vi "Set_Decoration_Color.vi"(0 "Pane ref":refnum<vi>, 5 "Data In":T1, 9 "Display State In":T2={"State 1"={"BG"=0, "FG"=0}, "State 0"={"BG"=0, "FG"=0}, "State 2"={"BG"=0, "FG"=0}, "State 3"={"BG"=0, "FG"=0}, "Shortcut Menu"=enum."Do left-click popup"}) -> ()   [LabVIEW 2011, in "Led.xctl"]
doc: "This VI changes the FG and BG colors of any decorations of the referenced VI pane in accordance with the Data In values."
uses:
  Led.xctl
  State.ctl
  TD_Status.ctl
panel:
  out "error out":errorcluster
  in  "error in":errorcluster
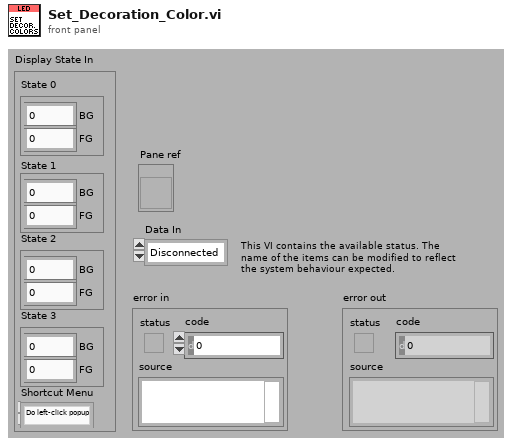
[diagram p1: front panel]
types:
  T1 = typedef "Led.xctl/TD_Status.ctl" = enum16{"Disconnected", "Connected", "Connecting", "Error"}
  T2 = typedef "Led.xctl/State.ctl" = cluster{"State 1":cluster{"BG":u32, "FG":u32}, "State 0":cluster{"BG":u32, "FG":u32}, "State 2":cluster{"BG":u32, "FG":u32}, "State 3":cluster{"BG":u32, "FG":u32}, "Shortcut Menu":enum16{"Treat normally", "Do left-click popup"}}
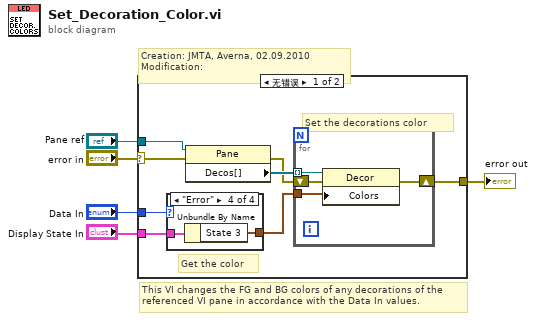
[diagram p0: block diagram]
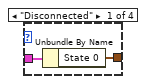
[diagram p2: hidden frame]
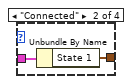
[diagram p3: hidden frame]
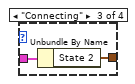
[diagram p4: hidden frame]
diagram:
  # "This VI changes the FG and BG colors of any decorations of the referenced VI pane in accordance with the Data In values."
  # "Creation: JMTA, Averna, 02.09.2010 \nModification:"
  n1 = case shown="无错误" "error in" {
    selector: "error in" -> [w7 w26]
    tunnel: "Display State In" -> [w11 _]
    tunnel: "Data In" -> [w10 _]
    tunnel: "Pane ref" -> [w8 _]
    tunnel: [w6 w26] -> w1
    frame No Error {
      # "Set the decorations color"
      # "Get the color"
      n2 = case shown="\"Error\"" w10 {
        tunnel: w11 -> [w15 w17 w19 w21]
        tunnel: [w14 w16 w18 w20] -> w12
        frame "Disconnected" {
          n3 = Unbundle By Name(w15) -> ("State 0"=w14:cluster{"BG":u32, "FG":u32})
        }
        frame "Connected" {
          n4 = Unbundle By Name(w17) -> ("State 1"=w16:cluster{"BG":u32, "FG":u32})
        }
        frame "Connecting" {
          n5 = Unbundle By Name(w19) -> ("State 2"=w18:cluster{"BG":u32, "FG":u32})
        }
        frame "Error" {
          n6 = Unbundle By Name(w21) -> ("State 3"=w20:cluster{"BG":u32, "FG":u32})
        }
      }
      n7 = property class="Pane"(reference=w8, error in=w7) -> (error out=w9:errorcluster, "Decos[]"=w13:refnum<vi>[])  [unwired: 1 out]
      n8 = for {
        tunnel: w13 -> [w25] mode=indexing
        tunnel: w12 -> [w24]
        shift-right: [w23] -> w6
        shift-left: w9 -> [w22]
        n9 = property class="Decor"(reference=w25, error in=w22, "Colors"=w24) -> (error out=w23:errorcluster)  [unwired: 1 out]
      }
    }
    frame Error {
    }
  }
  "error out" <- w1
